vi "ChainNode A.vi"(5 "Init State (\"Macro: Initialize\")":string="Macro: Initialize", 7 "Name (\"\" to Use UUID)":string="CSM-Module") -> ()   [LabVIEW 2017, in "Chain of Responsiblility Example.lvlib"]
uses:
  Chain of Responsiblility Example.lvlib
  user.lib/_NEVSTOP/Communicable State Machine(CSM)/AdvanceAPI/CSM - Revert Arguments-Safe String.vi
  user.lib/_NEVSTOP/Communicable State Machine(CSM)/AdvanceAPI/CSM - Make String Arguments Safe.vi
  user.lib/_NEVSTOP/Communicable State Machine(CSM)/AdvanceAPI/CSM - Break Down Multiple States String.vi
  user.lib/_NEVSTOP/Communicable State Machine(CSM)/AdvanceAPI/CSM - Compact Multiple States.vi
  user.lib/_NEVSTOP/Communicable State Machine(CSM)/AdvanceAPI/CSM - Keywords.vi
  user.lib/_NEVSTOP/Communicable State Machine(CSM)/_Shared/Trim Single-line Text.vi
  user.lib/_NEVSTOP/Communicable State Machine(CSM)/Communicable State Machine.lvlib
  user.lib/_NEVSTOP/Communicable State Machine(CSM)/_Shared/CSM Shared.lvlib
panel:
  out "Error Occurred":errorcluster
  out "State History":string
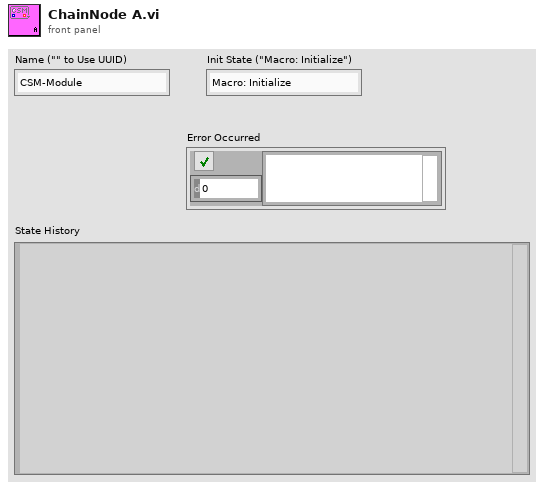
[diagram p1: front panel]
types:
  T1 = enum32{"Invalid", "Standard", "Closed", "Hidden", "Minimized", "Maximized"}
  T2 = enum32{"invalid app kind", "Development System", "Run Time System", "Student Edition", "Embedded LabVIEW", "Evaluation", "Custom"}
  T3 = typedef "Communicable State Machine.lvlib/_CSM_Response Source Message.ctl" = cluster{"‘State":string, "’Arguments":string, "’Error":errorcluster}
  T4 = cluster{"Current VI Reference":refnum<vi>, "Close Panel on Exit?":bool}
  T5 = cluster{"Core":cluster{"Current VI Reference":refnum<vi>, "Close Panel on Exit?":bool}, "Your Boolean data":bool, "Your string data":string}
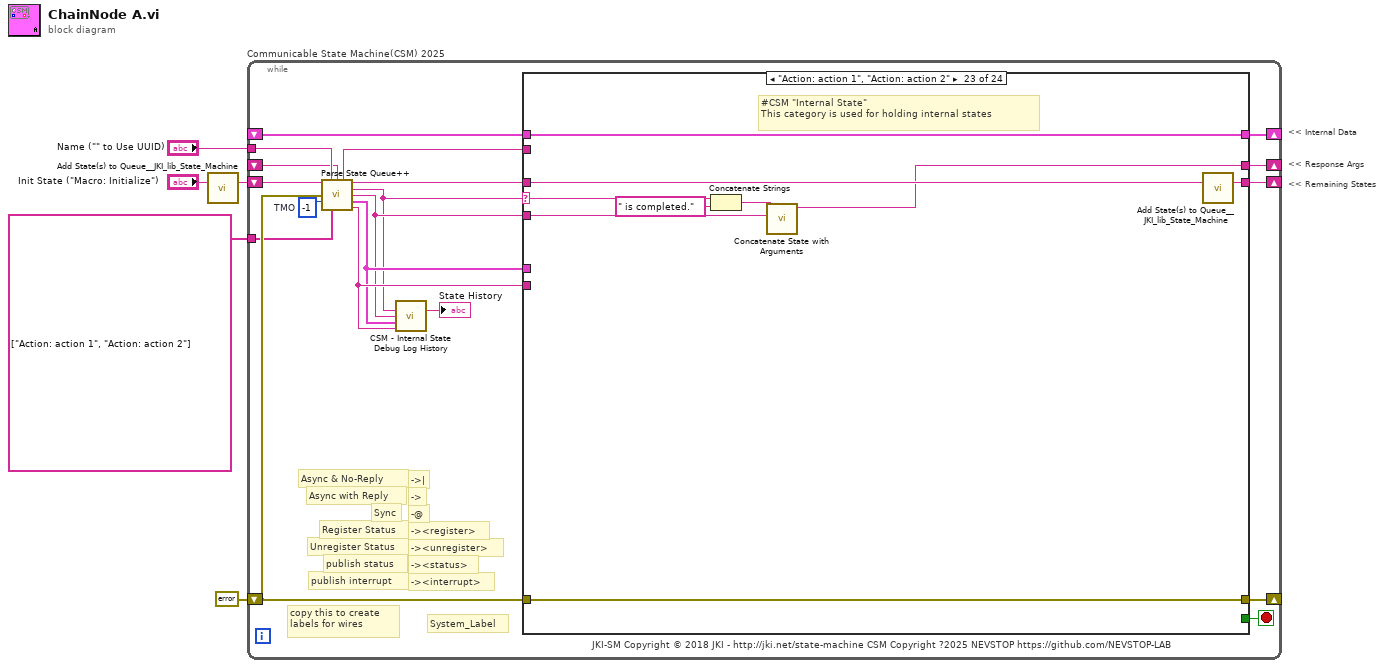
[diagram p0: block diagram]
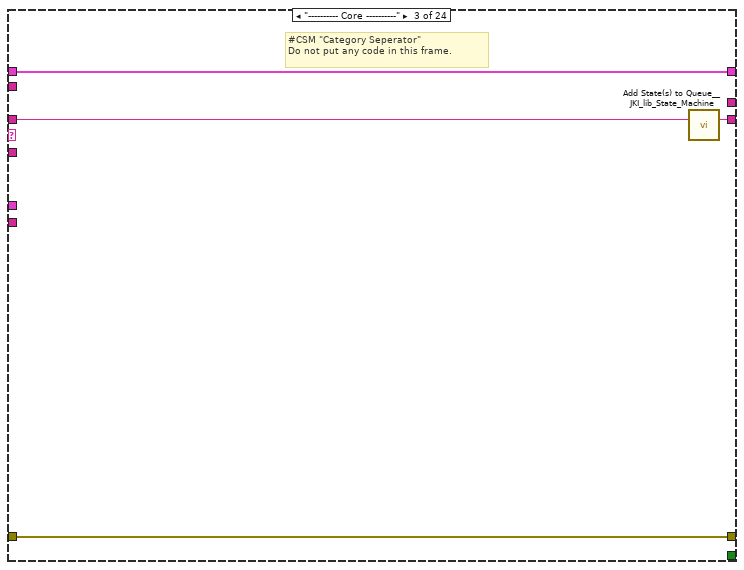
[diagram p4: hidden frame]
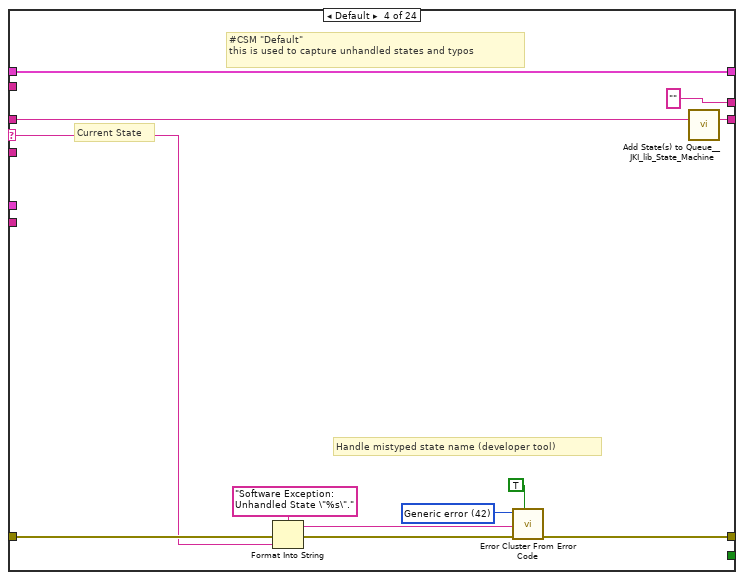
[diagram p5: hidden frame]
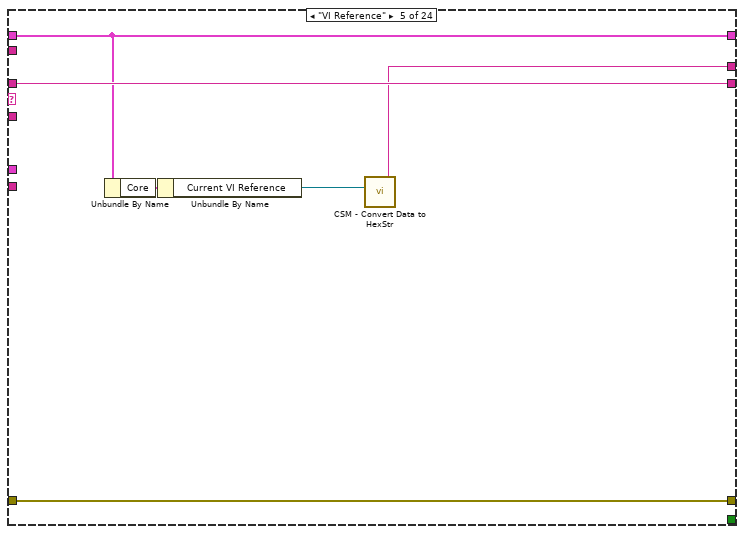
[diagram p6: hidden frame]
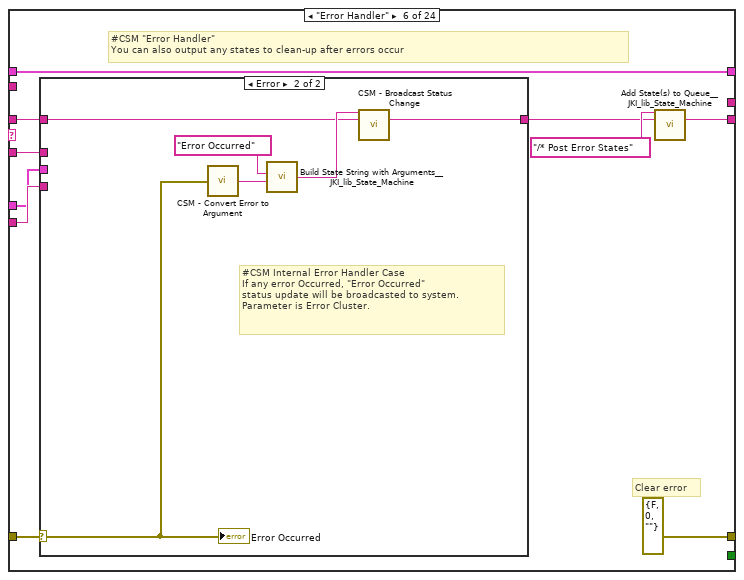
[diagram p7: hidden frame]
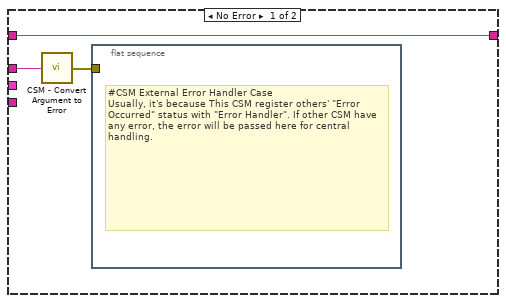
[diagram p8: hidden frame]
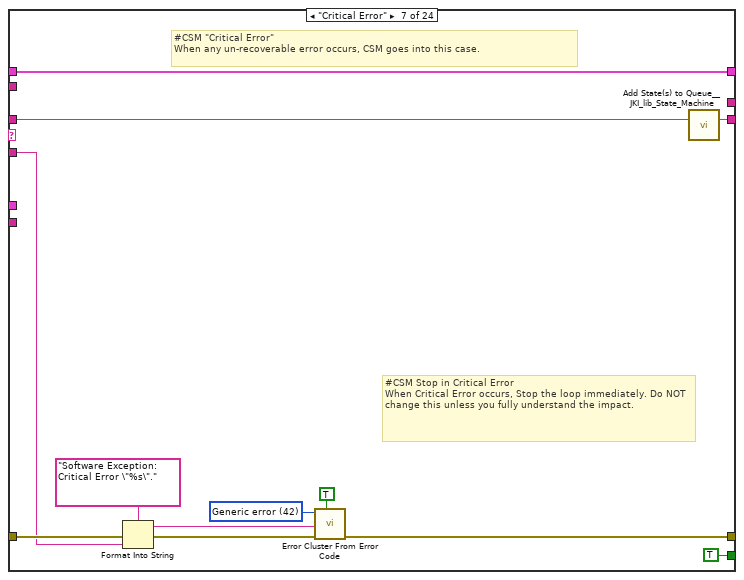
[diagram p9: hidden frame]
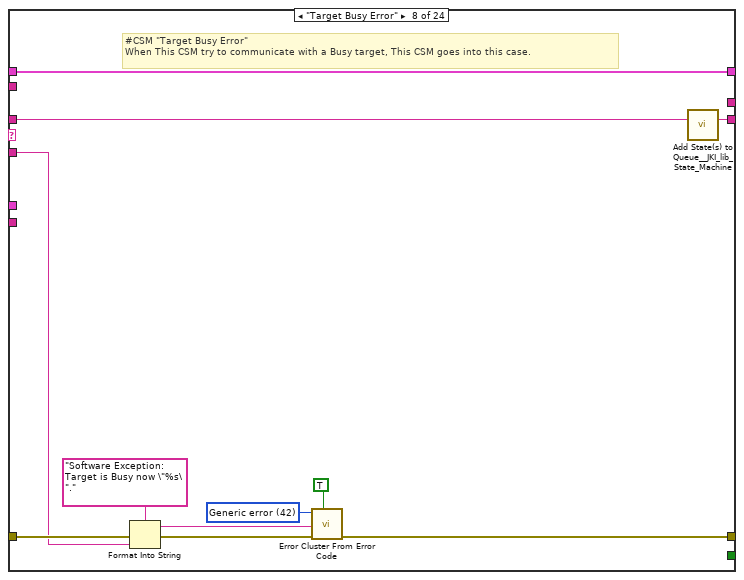
[diagram p10: hidden frame]
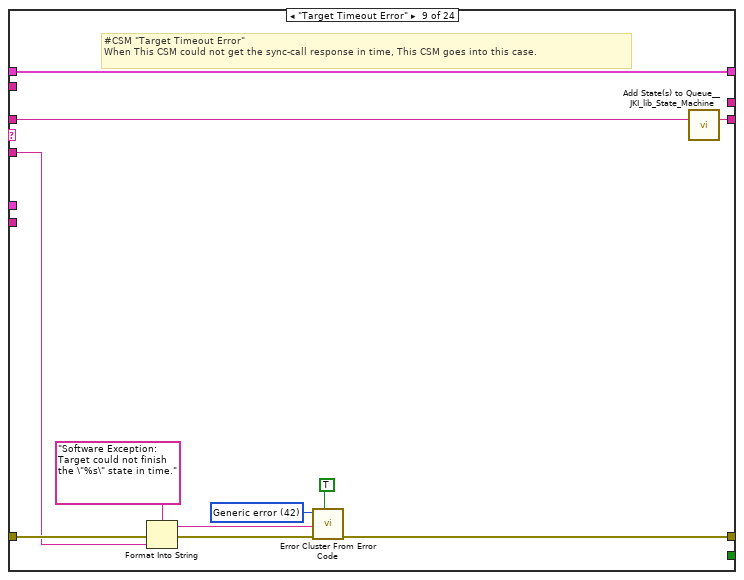
[diagram p11: hidden frame]
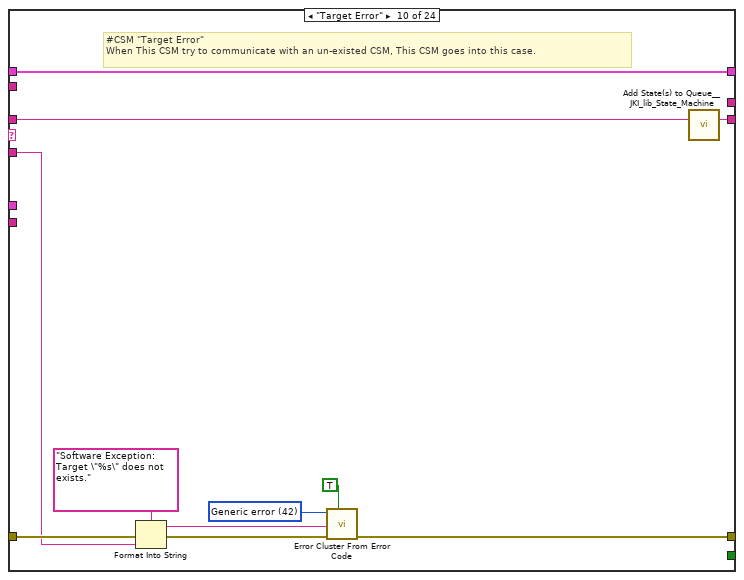
[diagram p12: hidden frame]
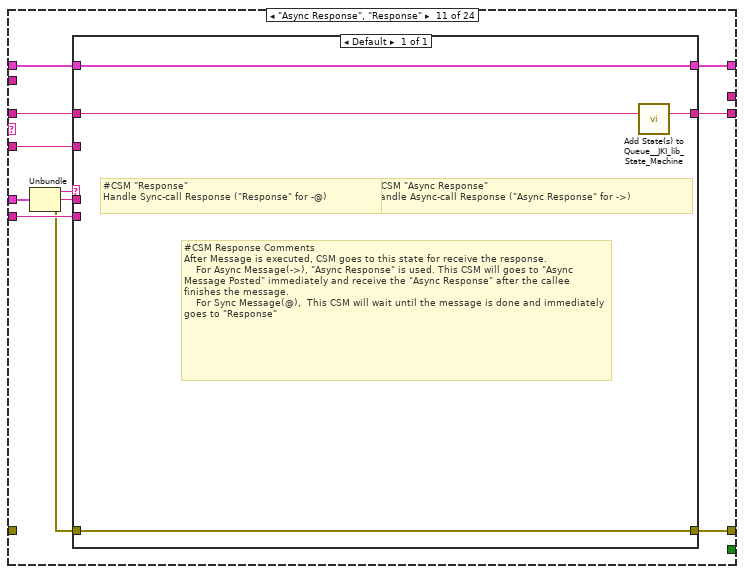
[diagram p13: hidden frame]
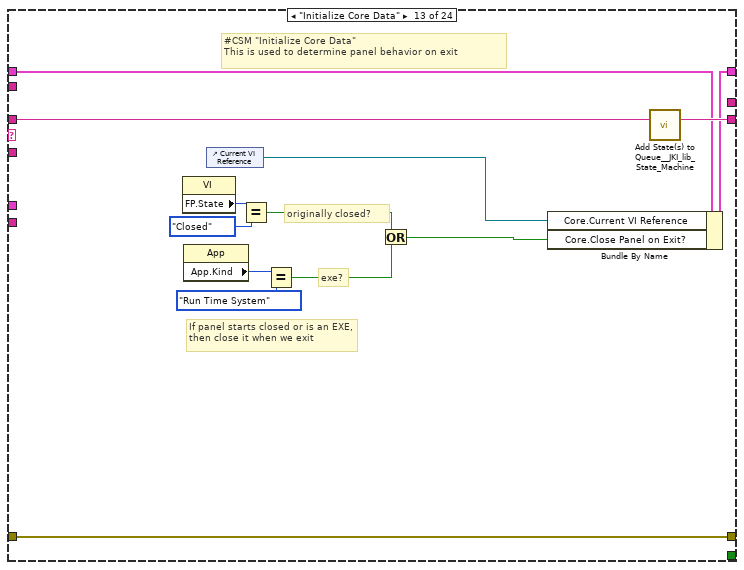
[diagram p15: hidden frame]
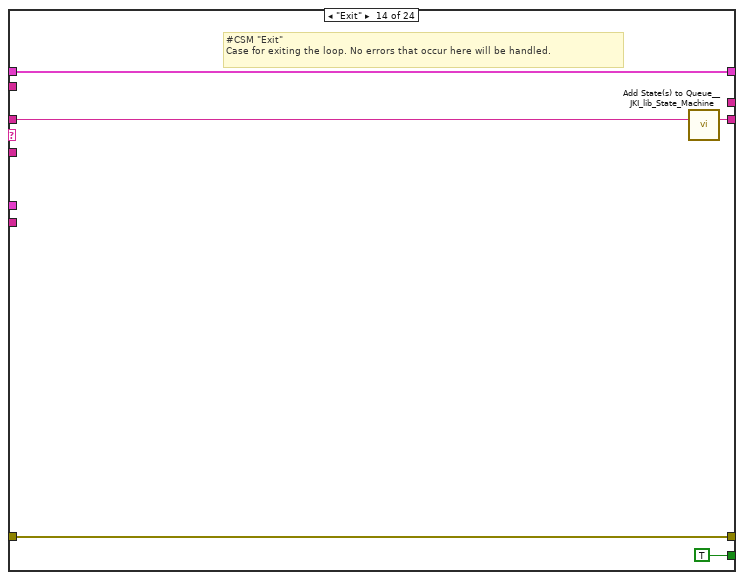
[diagram p16: hidden frame]
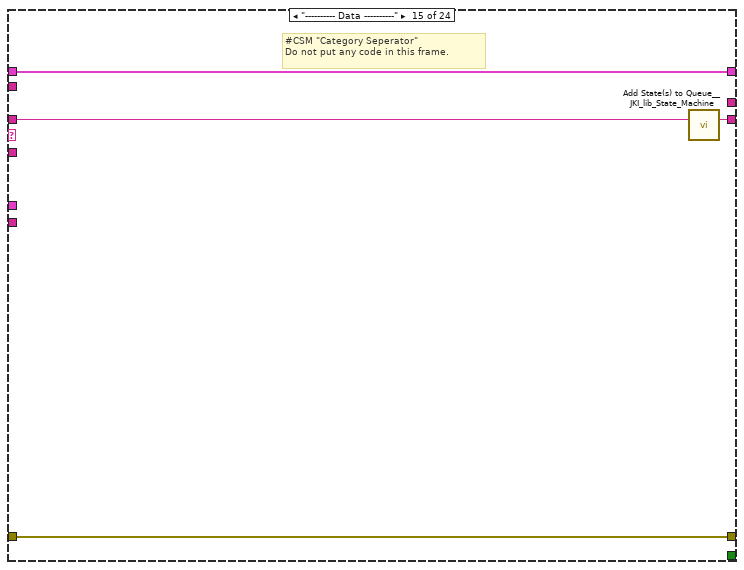
[diagram p17: hidden frame]
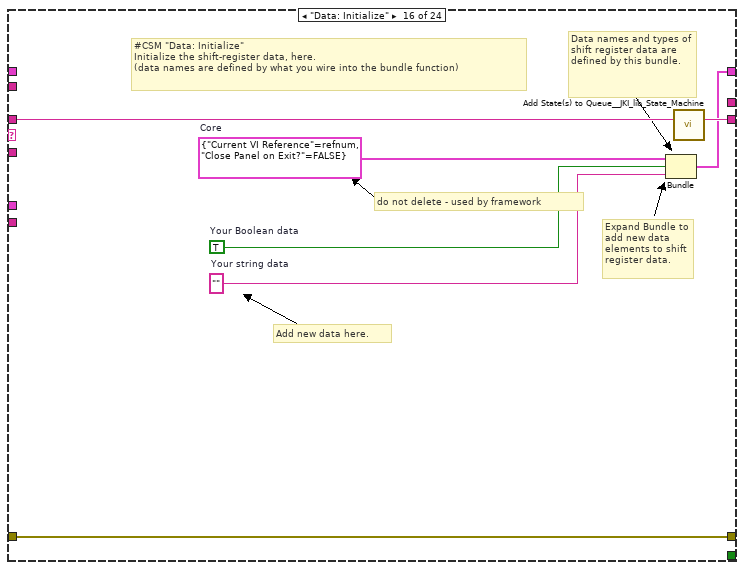
[diagram p18: hidden frame]
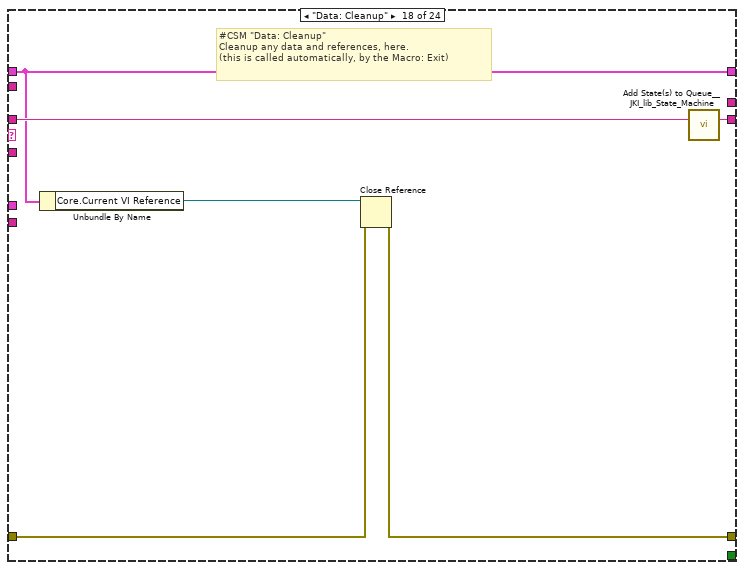
[diagram p20: hidden frame]
diagram:
  # "<< Internal Data"
  # "<< Response Args"
  # "<< Remaining States"
  n1 = call <vilib>:"Add State(s) to Queue__JKI_lib_State_Machine.vi"("State(s) in (\"\")"="Init State (\"Macro: Initialize\")") -> ("States Out"=w5:string)  [unwired: 14 in]
  n2 = while "Communicable State Machine(CSM) 2025" {
    shift-right: [w19] -> _
    shift-left: _ -> [w18]
    shift-right: [w22] -> _
    shift-left: errorcluster {"status"=FALSE, "code"=0, "source"=""} ("error out") -> [w8]
    shift-right: [w21] -> _
    shift-left: w5 -> [w23]
    tunnel: "Name (\"\" to Use UUID)" -> [w15]
    shift-right: [w16] -> _
    shift-left: _ -> [w10]
    tunnel: string[] ["Action: action 1", "Action: action 2"] ("Allowed Messages(Empty for all)") -> [w7]
    stop <- w20 stop-if-true
    w17 = -1  # TMO
    # "-><interrupt>"
    # "-><status>"
    # "-><unregister>"
    # "-><register>"
    # "-@"
    # "->"
    # "->|"
    # "publish interrupt"
    # "publish status"
    # "Unregister Status"
    # "Register Status"
    # "Sync"
    # "Async with Reply"
    # "Async & No-Reply"
    # "JKI-SM Copyright © 2018 JKI - http://jki.net/state-machine CSM Copyright ?2025 NEVSTOP https://github.com/NEVSTOP-LAB"
    # "copy this to create labels for wires"
    # "System_Label"
    n3 = call "Parse State Queue++.vi"("State Queue"=w23, "Name (\"\" to Use UUID)"=w15, "Response Arguments"=w10, "Previous Error"=w8, "Dequeue (1 ms)"=w17, "Allowed Messages (Empty for All)"=w7) -> ("Name Used"=w9:string, "Remaining States"=w24:string, "Current State"=w11:string, "Arguments"=w12:string, ">> Response Source Message >>"=w13:T3, ">> Source CSM >>"=w14:string)  [unwired: 4 in]
    n4 = call "CSM - Internal State Debug Log History.vi"("State"=w11, "Arguments (\"\")"=w12, ">> Response Source Message >>"=w13, "Source (\"\")"=w14) -> ("Debug Log"=→"State History":string)  [unwired: 11 in]
    n5 = case shown="\"Action: action 1\", \"Action: action 2\"" w11 {
      selector: w11 -> [_ _ _ w36 _ _ _ _ _ _ _ _ _ _ _ _ _ _ _ _ _ _ w195 _]
      tunnel: w24 -> [w25 w29 w34 w40 w51 w56 w77 w89 w100 w111 w126 w133 w147 w152 w156 w163 w165 w172 w176 w181 w186 w190 w199 w204]
      tunnel: w12 -> [_ _ _ _ _ w55 w73 w85 w96 w107 w120 _ _ _ _ _ _ _ _ _ _ _ w192 _]
      tunnel: w18 -> [w26 w28 w31 w38 w50 w61 w75 w87 w98 w109 w124 w132 w140 w150 w153 _ w164 w167 w173 w178 w183 w187 w196 w201]
      tunnel: [w27 w30 w32 w42 w52 errorcluster {"status"=FALSE, "code"=0, "source"=""} ("error out") w79 w84 w95 w106 w127 w134 w144 w149 w154 w160 w166 w168 w174 w179 w184 w188 w197 w202] -> w22
      tunnel: w8 -> [w27 w30 w32 w41 w52 w59 w78 w90 w101 w112 _ w134 w144 w149 w154 w160 w166 w169 w174 w179 w184 w188 w197 w202]
      tunnel: [w25 w29 w33 w39 w51 w57 w76 w88 w99 w110 w125 w133 w146 w151 w155 w162 w165 w171 w175 w180 w185 w189 w198 w203] -> w21
      tunnel: [_ _ _ _ _ _ TRUE _ _ _ _ _ _ TRUE _ _ _ _ _ _ _ _ _ _] -> w20
      tunnel: [w26 w28 w31 w38 w50 w61 w75 w87 w98 w109 w123 w132 w145 w150 w153 w161 w164 w167 w173 w178 w183 w187 w196 w201] -> w19
      tunnel: w14 -> [_ _ _ _ _ w54 _ _ _ _ w121 _ _ _ _ _ _ _ _ _ _ _ _ _]
      tunnel: w13 -> [_ _ _ _ _ w53 _ _ _ _ w122 _ _ _ _ _ _ _ _ _ _ _ _ _]
      tunnel: [_ _ _ "" w47 _ _ _ _ _ _ _ _ _ _ _ _ _ _ _ _ _ w191 "DoB Finished"] -> w16
      tunnel: w9 -> [_ _ _ _ _ _ _ _ _ _ _ _ _ _ _ _ _ _ _ _ _ _ _ _]
      frame "", "Idle" {
        # "#CSM \"Idle/Event Handler\"\nexecutes when the state queue is empty"
      }
      frame "CSM Documentation" {
        # "CSM Documentation"
        # "#CSM Commenting\nTo add a comment use \"//\" or \"#\" and all text to the right will be ignored\n\nCommenting Example:\nUI: Initialize // This initializes the UI\n// Another comment line"
        # "#CSM State Syntax\n\n    // Local Message Example\n    DoSth: DoA >> Arguments\n\n    // Sync Call Example\n    API: xxxx >> Arguments -@ TargetModule\n\n    // Async Call Example\n    API: xxxx >> Arguments -> TargetModule\n\n    // Async Call without Reply Example\n    API: xxxx >> Arguments ->| TargetModule\n\n    // Broadcast normal status:\n    Status >> StatusArguments  -><status>\n\n    // Broadcast Interrupt status:\n    Interrupt >> StatusArguments  -><interrupt>\n\n    // Register Source Module's status to Handler Module\n    Status@Source Module >> Handler Module@Handler Module -><register>\n\n    // Unegister Source Module's status\n    Status@Source Module >> Handler Module -><unregister>"
        # "#CSM README FIRST\n\nCSM is a LabVIEW application framework that builds upon JKI State Machine (CSM). It follows the pattern of CSM and extends the keywords to describe message communication between CSM modules, including concepts such as Sync-Message, Async-Message, Subscription/Unsubscription of status - essential elements for creating reusable code modules. For more information, please visit the CSM wiki: https://github.com/NEVSTOP-LAB/JKI-State-Machine-Plus-Plus/wiki\n\nFor instructions on JKI State Machine, visit: \n    http://jki.net/state-machine/\nFor information about CSM, visit: \n    https://github.com/NEVSTOP-LAB"
        # "#CSM \"Documentation\"\nCase for holding CSM Documenation"
      }
      frame "---------- Core ----------" {
        # "#CSM \"Category Seperator\"\nDo not put any code in this frame."
        n6 = call <vilib>:"Add State(s) to Queue__JKI_lib_State_Machine.vi"("State(s) in (\"\")"=w34) -> ("States Out"=w33:string)  [unwired: 14 in]
      }
      frame Default {
        w45 = 42 items=["No error", "Argument error", "Memory is full", "Out of zone", "End of file", "File already open", "Generic file I/O error", "File not found", "File permission error", "Disk is full", "Duplicate path", "Too many files open", "System feature not enabled", "Resource file not found", "Cannot add resource", "Resource not found", "Image not found", "Image memory error", "Pen does not exist", "Config type invalid", "Config token not found", "Config parse error", "Config memory error", "Bad external code format", "Bad external code offset", "External code not present", "Null window", "Destroy window error", "Null menu", "Print aborted", "Bad print record", "Print driver error", "Windows error during printing", "Memory error during printing", "Print dialog error", "Generic print error", "Invalid device refnum", "Device not found", "Device parameter error", "Device unit error", "Cannot open device", "Device call aborted", "Generic error", "Cancelled by user", "Object ID too low", "Object ID too high", "Object not in heap", "Unknown heap", "Unknown object (invalid DefProc)", "Unknown object (DefProc not in table)", "Message out of range", "Invalid (null) method", "Unknown message", "Manager call not supported", "Bad address", "Network operation in progress", "Network operation timed out", "Connection is busy", "Network attribute not supported", "Network error", "Address in use", "System out of memory", "Connection aborted", "Connection refused", "Not connected", "Already connected", "Connection closed", "Initialization error (interapplication manager)", "Bad occurrence", "Wait on unbound occurrence handler", "Occurrence queue overflow", "Datalog type conflict", "Unused", "Unrecognized type (interapplication manager)", "Memory corrupt", "Failed to make temporary DLL", "Old CIN version", "Drag socket not found", "Failed to load drop-object", "Failed to register OLE object", "Failed to release OLE object", "Format specifier type mismatch", "Unknown format specifier", "Too few format specifiers", "Too many format specifiers", "Scan failed", "Newer CIN version", "Error converting to variant", "Runtime menu error", "Password tampered", "Variant attribute not found", "Incompatible variant data type", "Event data is not available", "Event Store is not present", "Occurrence is not found", "Event Queue is not created", "Event info is not available", "Refnum passed is NULL", "Error retrieving Class GUID", "Error retrieving CoClass GUID", "Error retrieving TypeLib GUID.", "Bad built application magic bytes.", "Specific driver is different from the specific driver associated with the Logical Name.", "There is no session opened to the class driver.", "Max Error", "MAX - Error with config objects", "MAX - Error loading configuration", "MAX - Group not supported"]
        # "#CSM \"Default\"\nthis is used to capture unhandled states and typos"
        # "Current State"
        # "Handle mistyped state name (developer tool)"
        n7 = Format Into String(format string="Software Exception: Unhandled State \"%s\"." ("message"), error in=w41, w36) -> (resulting string=w44:string, error out=w43:errorcluster)  [unwired: 1 in]
        n8 = call <vilib>:"Error Cluster From Error Code.vi"("show call chain? (False)"=TRUE, "error in (no error)"=w43, "error message (\"\")"=w44, "error code (0)"=w45) -> ("error out"=w42:errorcluster)  [unwired: 5 in]
        n9 = call <vilib>:"Add State(s) to Queue__JKI_lib_State_Machine.vi"("State(s) in (\"\")"=w40) -> ("States Out"=w39:string)  [unwired: 14 in]
      }
      frame "VI Reference" {
        n10 = Unbundle By Name(w50) -> ("Core"=w49:T4)
        n11 = Unbundle By Name(w49) -> ("Current VI Reference"=w48:refnum<vi>)
        n12 = call "CSM - Convert Data to HexStr.vi"("Variant"=w48) -> ("HEX String (0-9,A-F)"=w47:string)  [unwired: 8 in]
      }
      frame "Error Handler" {
        # "#CSM \"Error Handler\"\nYou can also output any states to clean-up after errors occur"
        # "Clear error"
        n13 = case shown="Error" w59 {
          selector: w59 -> [_ w66]
          tunnel: [w65 w68] -> w58
          tunnel: w56 -> [w65 w67]
          tunnel: w55 -> [w64 _]
          tunnel: w54 -> [_ _]
          tunnel: w53 -> [_ _]
          frame No Error {
            n14 = call "CSM - Convert Argument to Error.vi"("Argument"=w64) -> ("Error"=w63:errorcluster)  [unwired: 4 in]
            n15 = flat-sequence {
              tunnel: w63 -> [_]
              frame #0 {
                # "#CSM External Error Handler Case\nUsually, it's because This CSM register others' \"Error Occurred\" status with \"Error Handler\". If other CSM have any error, the error will be passed here for central handling."
              }
            }
          }
          frame Error {
            # "#CSM Internal Error Handler Case \nIf any error Occurred, \"Error Occurred\" \nstatus update will be broadcasted to system.\nParameter is Error Cluster."
            n16 = call "CSM - Convert Error to Argument.vi"("Error"=w66) -> ("Argument"=w70:string)  [unwired: 4 in]
            n17 = call <vilib>:"Build State String with Arguments__JKI_lib_State_Machine.vi"("Arguments (\"\")"=w70, "State"="Error Occurred" ("Status with Arguments")) -> ("State with Arguments"=w69:string)  [unwired: 4 in]
            n18 = call "CSM - Broadcast Status Change.vi"("Status With Arguments"=w69, "State Queue"=w67) -> ("Remaining States"=w68:string)  [unwired: 13 in]
            "Error Occurred" <- w66
          }
        }
        n19 = call <vilib>:"Add State(s) to Queue__JKI_lib_State_Machine.vi"("State(s) in Front (\"\")"="/* Post Error States", "State(s) in (\"\")"=w58) -> ("States Out"=w57:string)  [unwired: 13 in]
      }
      frame "Critical Error" {
        w82 = 42 items=["No error", "Argument error", "Memory is full", "Out of zone", "End of file", "File already open", "Generic file I/O error", "File not found", "File permission error", "Disk is full", "Duplicate path", "Too many files open", "System feature not enabled", "Resource file not found", "Cannot add resource", "Resource not found", "Image not found", "Image memory error", "Pen does not exist", "Config type invalid", "Config token not found", "Config parse error", "Config memory error", "Bad external code format", "Bad external code offset", "External code not present", "Null window", "Destroy window error", "Null menu", "Print aborted", "Bad print record", "Print driver error", "Windows error during printing", "Memory error during printing", "Print dialog error", "Generic print error", "Invalid device refnum", "Device not found", "Device parameter error", "Device unit error", "Cannot open device", "Device call aborted", "Generic error", "Cancelled by user", "Object ID too low", "Object ID too high", "Object not in heap", "Unknown heap", "Unknown object (invalid DefProc)", "Unknown object (DefProc not in table)", "Message out of range", "Invalid (null) method", "Unknown message", "Manager call not supported", "Bad address", "Network operation in progress", "Network operation timed out", "Connection is busy", "Network attribute not supported", "Network error", "Address in use", "System out of memory", "Connection aborted", "Connection refused", "Not connected", "Already connected", "Connection closed", "Initialization error (interapplication manager)", "Bad occurrence", "Wait on unbound occurrence handler", "Occurrence queue overflow", "Datalog type conflict", "Unused", "Unrecognized type (interapplication manager)", "Memory corrupt", "Failed to make temporary DLL", "Old CIN version", "Drag socket not found", "Failed to load drop-object", "Failed to register OLE object", "Failed to release OLE object", "Format specifier type mismatch", "Unknown format specifier", "Too few format specifiers", "Too many format specifiers", "Scan failed", "Newer CIN version", "Error converting to variant", "Runtime menu error", "Password tampered", "Variant attribute not found", "Incompatible variant data type", "Event data is not available", "Event Store is not present", "Occurrence is not found", "Event Queue is not created", "Event info is not available", "Refnum passed is NULL", "Error retrieving Class GUID", "Error retrieving CoClass GUID", "Error retrieving TypeLib GUID.", "Bad built application magic bytes.", "Specific driver is different from the specific driver associated with the Logical Name.", "There is no session opened to the class driver.", "Max Error", "MAX - Error with config objects", "MAX - Error loading configuration", "MAX - Group not supported"]
        # "#CSM \"Critical Error\"\nWhen any un-recoverable error occurs, CSM goes into this case."
        # "#CSM Stop in Critical Error\nWhen Critical Error occurs, Stop the loop immediately. Do NOT change this unless you fully understand the impact."
        n20 = Format Into String(format string="Software Exception: Critical Error \"%s\"." ("message"), error in=w78, w73) -> (resulting string=w81:string, error out=w80:errorcluster)  [unwired: 1 in]
        n21 = call <vilib>:"Error Cluster From Error Code.vi"("show call chain? (False)"=TRUE, "error in (no error)"=w80, "error message (\"\")"=w81, "error code (0)"=w82) -> ("error out"=w79:errorcluster)  [unwired: 5 in]
        n22 = call <vilib>:"Add State(s) to Queue__JKI_lib_State_Machine.vi"("State(s) in (\"\")"=w77) -> ("States Out"=w76:string)  [unwired: 14 in]
      }
      frame "Target Busy Error" {
        w93 = 42 items=["No error", "Argument error", "Memory is full", "Out of zone", "End of file", "File already open", "Generic file I/O error", "File not found", "File permission error", "Disk is full", "Duplicate path", "Too many files open", "System feature not enabled", "Resource file not found", "Cannot add resource", "Resource not found", "Image not found", "Image memory error", "Pen does not exist", "Config type invalid", "Config token not found", "Config parse error", "Config memory error", "Bad external code format", "Bad external code offset", "External code not present", "Null window", "Destroy window error", "Null menu", "Print aborted", "Bad print record", "Print driver error", "Windows error during printing", "Memory error during printing", "Print dialog error", "Generic print error", "Invalid device refnum", "Device not found", "Device parameter error", "Device unit error", "Cannot open device", "Device call aborted", "Generic error", "Cancelled by user", "Object ID too low", "Object ID too high", "Object not in heap", "Unknown heap", "Unknown object (invalid DefProc)", "Unknown object (DefProc not in table)", "Message out of range", "Invalid (null) method", "Unknown message", "Manager call not supported", "Bad address", "Network operation in progress", "Network operation timed out", "Connection is busy", "Network attribute not supported", "Network error", "Address in use", "System out of memory", "Connection aborted", "Connection refused", "Not connected", "Already connected", "Connection closed", "Initialization error (interapplication manager)", "Bad occurrence", "Wait on unbound occurrence handler", "Occurrence queue overflow", "Datalog type conflict", "Unused", "Unrecognized type (interapplication manager)", "Memory corrupt", "Failed to make temporary DLL", "Old CIN version", "Drag socket not found", "Failed to load drop-object", "Failed to register OLE object", "Failed to release OLE object", "Format specifier type mismatch", "Unknown format specifier", "Too few format specifiers", "Too many format specifiers", "Scan failed", "Newer CIN version", "Error converting to variant", "Runtime menu error", "Password tampered", "Variant attribute not found", "Incompatible variant data type", "Event data is not available", "Event Store is not present", "Occurrence is not found", "Event Queue is not created", "Event info is not available", "Refnum passed is NULL", "Error retrieving Class GUID", "Error retrieving CoClass GUID", "Error retrieving TypeLib GUID.", "Bad built application magic bytes.", "Specific driver is different from the specific driver associated with the Logical Name.", "There is no session opened to the class driver.", "Max Error", "MAX - Error with config objects", "MAX - Error loading configuration", "MAX - Group not supported"]
        # "#CSM \"Target Busy Error\"\nWhen This CSM try to communicate with a Busy target, This CSM goes into this case."
        n23 = Format Into String(format string="Software Exception: Target is Busy now \"%s\"." ("message"), error in=w90, w85) -> (resulting string=w92:string, error out=w91:errorcluster)  [unwired: 1 in]
        n24 = call <vilib>:"Error Cluster From Error Code.vi"("show call chain? (False)"=TRUE, "error in (no error)"=w91, "error message (\"\")"=w92, "error code (0)"=w93) -> ("error out"=w84:errorcluster)  [unwired: 5 in]
        n25 = call <vilib>:"Add State(s) to Queue__JKI_lib_State_Machine.vi"("State(s) in (\"\")"=w89) -> ("States Out"=w88:string)  [unwired: 14 in]
      }
      frame "Target Timeout Error" {
        w104 = 42 items=["No error", "Argument error", "Memory is full", "Out of zone", "End of file", "File already open", "Generic file I/O error", "File not found", "File permission error", "Disk is full", "Duplicate path", "Too many files open", "System feature not enabled", "Resource file not found", "Cannot add resource", "Resource not found", "Image not found", "Image memory error", "Pen does not exist", "Config type invalid", "Config token not found", "Config parse error", "Config memory error", "Bad external code format", "Bad external code offset", "External code not present", "Null window", "Destroy window error", "Null menu", "Print aborted", "Bad print record", "Print driver error", "Windows error during printing", "Memory error during printing", "Print dialog error", "Generic print error", "Invalid device refnum", "Device not found", "Device parameter error", "Device unit error", "Cannot open device", "Device call aborted", "Generic error", "Cancelled by user", "Object ID too low", "Object ID too high", "Object not in heap", "Unknown heap", "Unknown object (invalid DefProc)", "Unknown object (DefProc not in table)", "Message out of range", "Invalid (null) method", "Unknown message", "Manager call not supported", "Bad address", "Network operation in progress", "Network operation timed out", "Connection is busy", "Network attribute not supported", "Network error", "Address in use", "System out of memory", "Connection aborted", "Connection refused", "Not connected", "Already connected", "Connection closed", "Initialization error (interapplication manager)", "Bad occurrence", "Wait on unbound occurrence handler", "Occurrence queue overflow", "Datalog type conflict", "Unused", "Unrecognized type (interapplication manager)", "Memory corrupt", "Failed to make temporary DLL", "Old CIN version", "Drag socket not found", "Failed to load drop-object", "Failed to register OLE object", "Failed to release OLE object", "Format specifier type mismatch", "Unknown format specifier", "Too few format specifiers", "Too many format specifiers", "Scan failed", "Newer CIN version", "Error converting to variant", "Runtime menu error", "Password tampered", "Variant attribute not found", "Incompatible variant data type", "Event data is not available", "Event Store is not present", "Occurrence is not found", "Event Queue is not created", "Event info is not available", "Refnum passed is NULL", "Error retrieving Class GUID", "Error retrieving CoClass GUID", "Error retrieving TypeLib GUID.", "Bad built application magic bytes.", "Specific driver is different from the specific driver associated with the Logical Name.", "There is no session opened to the class driver.", "Max Error", "MAX - Error with config objects", "MAX - Error loading configuration", "MAX - Group not supported"]
        # "#CSM \"Target Timeout Error\"\nWhen This CSM could not get the sync-call response in time, This CSM goes into this case."
        n26 = Format Into String(format string="Software Exception: Target could not finish the \"%s\" state in time." ("message"), error in=w101, w96) -> (resulting string=w103:string, error out=w102:errorcluster)  [unwired: 1 in]
        n27 = call <vilib>:"Error Cluster From Error Code.vi"("show call chain? (False)"=TRUE, "error in (no error)"=w102, "error message (\"\")"=w103, "error code (0)"=w104) -> ("error out"=w95:errorcluster)  [unwired: 5 in]
        n28 = call <vilib>:"Add State(s) to Queue__JKI_lib_State_Machine.vi"("State(s) in (\"\")"=w100) -> ("States Out"=w99:string)  [unwired: 14 in]
      }
      frame "Target Error" {
        w115 = 42 items=["No error", "Argument error", "Memory is full", "Out of zone", "End of file", "File already open", "Generic file I/O error", "File not found", "File permission error", "Disk is full", "Duplicate path", "Too many files open", "System feature not enabled", "Resource file not found", "Cannot add resource", "Resource not found", "Image not found", "Image memory error", "Pen does not exist", "Config type invalid", "Config token not found", "Config parse error", "Config memory error", "Bad external code format", "Bad external code offset", "External code not present", "Null window", "Destroy window error", "Null menu", "Print aborted", "Bad print record", "Print driver error", "Windows error during printing", "Memory error during printing", "Print dialog error", "Generic print error", "Invalid device refnum", "Device not found", "Device parameter error", "Device unit error", "Cannot open device", "Device call aborted", "Generic error", "Cancelled by user", "Object ID too low", "Object ID too high", "Object not in heap", "Unknown heap", "Unknown object (invalid DefProc)", "Unknown object (DefProc not in table)", "Message out of range", "Invalid (null) method", "Unknown message", "Manager call not supported", "Bad address", "Network operation in progress", "Network operation timed out", "Connection is busy", "Network attribute not supported", "Network error", "Address in use", "System out of memory", "Connection aborted", "Connection refused", "Not connected", "Already connected", "Connection closed", "Initialization error (interapplication manager)", "Bad occurrence", "Wait on unbound occurrence handler", "Occurrence queue overflow", "Datalog type conflict", "Unused", "Unrecognized type (interapplication manager)", "Memory corrupt", "Failed to make temporary DLL", "Old CIN version", "Drag socket not found", "Failed to load drop-object", "Failed to register OLE object", "Failed to release OLE object", "Format specifier type mismatch", "Unknown format specifier", "Too few format specifiers", "Too many format specifiers", "Scan failed", "Newer CIN version", "Error converting to variant", "Runtime menu error", "Password tampered", "Variant attribute not found", "Incompatible variant data type", "Event data is not available", "Event Store is not present", "Occurrence is not found", "Event Queue is not created", "Event info is not available", "Refnum passed is NULL", "Error retrieving Class GUID", "Error retrieving CoClass GUID", "Error retrieving TypeLib GUID.", "Bad built application magic bytes.", "Specific driver is different from the specific driver associated with the Logical Name.", "There is no session opened to the class driver.", "Max Error", "MAX - Error with config objects", "MAX - Error loading configuration", "MAX - Group not supported"]
        # "#CSM \"Target Error\"\nWhen This CSM try to communicate with an un-existed CSM, This CSM goes into this case."
        n29 = Format Into String(format string="Software Exception: Target \"%s\" does not exists." ("message"), error in=w112, w107) -> (resulting string=w114:string, error out=w113:errorcluster)  [unwired: 1 in]
        n30 = call <vilib>:"Error Cluster From Error Code.vi"("show call chain? (False)"=TRUE, "error in (no error)"=w113, "error message (\"\")"=w114, "error code (0)"=w115) -> ("error out"=w106:errorcluster)  [unwired: 5 in]
        n31 = call <vilib>:"Add State(s) to Queue__JKI_lib_State_Machine.vi"("State(s) in (\"\")"=w111) -> ("States Out"=w110:string)  [unwired: 14 in]
      }
      frame "Async Response", "Response" {
        n32 = Unbundle(w122) -> ("‘State"=w119:string, "’Arguments"=w118:string, "’Error"=w117:errorcluster)
        n33 = case shown="Default" w119 {
          tunnel: [w128] -> w125
          tunnel: w126 -> [w129]
          tunnel: [w131] -> w123
          tunnel: w124 -> [w131]
          tunnel: [w130] -> w127
          tunnel: w117 -> [w130]
          tunnel: w121 -> [_]
          tunnel: w120 -> [_]
          tunnel: w118 -> [_]
          frame Default {
            # "#CSM \"Async Response\"\nHandle Async-call Response (\"Async Response\" for ->)"
            # "#CSM \"Response\"\nHandle Sync-call Response (\"Response\" for -@)"
            # "#CSM Response Comments\nAfter Message is executed, CSM goes to this state for receive the response.\n    For Async Message(->), \"Async Response\" is used. This CSM will goes to \"Async Message Posted\" immediately and receive the \"Async Response\" after the callee finishes the message.\n    For Sync Message(@),  This CSM will wait until the message is done and immediately goes to \"Response\""
            n34 = call <vilib>:"Add State(s) to Queue__JKI_lib_State_Machine.vi"("State(s) in (\"\")"=w129) -> ("States Out"=w128:string)  [unwired: 14 in]
          }
        }
      }
      frame "Async Message Posted" {
        # "#CSM \"Async Message Posted\"\nAfter Async Message is posted (-> or ->| ), CSM goes to this state for post-action.\nYou can use Argument - State to tell which Async Message is called."
      }
      frame "Initialize Core Data" {
        # "#CSM \"Initialize Core Data\"\nThis is used to determine panel behavior on exit"
        # "originally closed?"
        # "exe?"
        # "If panel starts closed or is an EXE, then close it when we exit"
        n35 = property class="VI"() -> ("FP.State"=w137:T1)  [unwired: 2 in, 2 out]
        n36 = property class="App"() -> ("App.Kind"=w143:T2)  [unwired: 2 in, 2 out]
        n37 = control-ref of="Current VI Reference"() -> (w138:refnum<vi>)
        n38 = Equal?(x=w137, y=T1."Closed" ("Front Panel Window:State")) -> (x = y?=w135:bool)
        n39 = Equal?(x=w143, y=T2."Run Time System" ("Application:Kind")) -> (x = y?=w141:bool)
        n40 = Or(x=w135, y=w141) -> (x .or. y?=w139:bool)
        n41 = Bundle By Name(cluster=w140, "Core.Current VI Reference"=w138, "Core.Close Panel on Exit?"=w139) -> (w145:T5)
        n42 = call <vilib>:"Add State(s) to Queue__JKI_lib_State_Machine.vi"("State(s) in (\"\")"=w147) -> ("States Out"=w146:string)  [unwired: 14 in]
      }
      frame "Exit" {
        # "#CSM \"Exit\"\nCase for exiting the loop. No errors that occur here will be handled."
        n43 = call <vilib>:"Add State(s) to Queue__JKI_lib_State_Machine.vi"("State(s) in (\"\")"=w152) -> ("States Out"=w151:string)  [unwired: 14 in]
      }
      frame "---------- Data ----------" {
        # "#CSM \"Category Seperator\"\nDo not put any code in this frame."
        n44 = call <vilib>:"Add State(s) to Queue__JKI_lib_State_Machine.vi"("State(s) in (\"\")"=w156) -> ("States Out"=w155:string)  [unwired: 14 in]
      }
      frame "Data: Initialize" {
        w157 = T4 {"Current VI Reference"=refnum, "Close Panel on Exit?"=FALSE}  # Core
        w159 = TRUE  # Your Boolean data
        w158 = ""  # Your string data
        # "#CSM \"Data: Initialize\"\nInitialize the shift-register data, here.\n(data names are defined by what you wire into the bundle function)"
        # "do not delete - used by framework"
        # "Expand Bundle to add new data elements to shift register data."
        # "Add new data here."
        # "Data names and types of shift register data are defined by this bundle."
        n45 = Bundle("Core"=w157, "Your Boolean data"=w159, "Your string data"=w158) -> (w161:T5)  [unwired: 1 in]
        n46 = call <vilib>:"Add State(s) to Queue__JKI_lib_State_Machine.vi"("State(s) in (\"\")"=w163) -> ("States Out"=w162:string)  [unwired: 14 in]
      }
      frame "Data: Update Indicators" {
      }
      frame "Data: Cleanup" {
        # "#CSM \"Data: Cleanup\"\nCleanup any data and references, here.\n(this is called automatically, by the Macro: Exit)"
        n47 = Unbundle By Name(w167) -> ("Core.Current VI Reference"=w170:refnum<vi>)
        n48 = Close Reference(reference=w170, error in (no error)=w169) -> (error out=w168:errorcluster)
        n49 = call <vilib>:"Add State(s) to Queue__JKI_lib_State_Machine.vi"("State(s) in (\"\")"=w172) -> ("States Out"=w171:string)  [unwired: 14 in]
      }
      frame "---------- Macro ----------" {
        # "#CSM \"Category Seperator\"\nDo not put any code in this frame."
        n50 = call <vilib>:"Add State(s) to Queue__JKI_lib_State_Machine.vi"("State(s) in (\"\")"=w176) -> ("States Out"=w175:string)  [unwired: 14 in]
      }
      frame "Macro: Initialize" {
        # "#CSM \"Macro: Initialize\"\nInitialization Macro (This is called once, when the VI starts)"
        n51 = call <vilib>:"Add State(s) to Queue__JKI_lib_State_Machine.vi"("State(s) in Front (\"\")"="Data: Initialize\nInitialize Core Data\nData: Update Indicators", "State(s) in (\"\")"=w181) -> ("States Out"=w180:string)  [unwired: 13 in]
      }
      frame "Macro: Exit" {
        # "#CSM \"Macro: Exit\"\nExit Macro (This is called once, when the VI exits)"
        n52 = call <vilib>:"Add State(s) to Queue__JKI_lib_State_Machine.vi"("State(s) in Front (\"\")"="Data: Cleanup\nExit", "State(s) in (\"\")"=w186) -> ("States Out"=w185:string)  [unwired: 13 in]
      }
      frame "---------- DoSth ----------" {
        # "#CSM \"Category Seperator\"\nDo not put any code in this frame."
        n53 = call <vilib>:"Add State(s) to Queue__JKI_lib_State_Machine.vi"("State(s) in (\"\")"=w190) -> ("States Out"=w189:string)  [unwired: 14 in]
      }
      frame "Action: action 1", "Action: action 2" {
        # "#CSM \"Internal State\"\nThis category is used for holding internal states"
        n54 = Concatenate Strings(w195, " is completed." ("string")) -> (w193:string)
        n55 = call "Concatenate State with Arguments.vi"("Arguments"=w192, "State"=w193) -> ("State With Arguements"=w191:string)  [unwired: 9 in]
        n56 = call <vilib>:"Add State(s) to Queue__JKI_lib_State_Machine.vi"("State(s) in (\"\")"=w199) -> ("States Out"=w198:string)  [unwired: 14 in]
      }
      frame "DoSth: DoB" {
        # "#CSM \"Internal State\"\nThis category is used for holding internal states"
        n57 = call <vilib>:"Add State(s) to Queue__JKI_lib_State_Machine.vi"("State(s) in (\"\")"=w204) -> ("States Out"=w203:string)  [unwired: 14 in]
      }
    }
  }
